vi "Noise_meas.vi"() -> ()   [LabVIEW 2013]
uses:
  <vilib>/DAQmx/read.llb/DAQmx Read (Analog 2D DBL NChan NSamp).vi
  <vilib>/DAQmx/create/channels.llb/DAQmx Create Channel (AI-Voltage-Basic).vi
  <vilib>/DAQmx/configure/timing.llb/DAQmx Timing (Sample Clock).vi
  <vilib>/Analysis/2dsp.llb/1D Cross Correlation (DBL).vi
  <vilib>/DAQmx/miscellaneous.llb/DAQmx Fill In Error Info.vi
  <vilib>/express/express analysis/Spectral/Block/exnSpectralBlock spectral measurements RMS poly.vi
  <vilib>/express/express analysis/Spectral/Block/exnSpectralBlock spectral measurements RMS WFM.vi
  <vilib>/express/express analysis/Spectral/Block/exnSpectralBlock spectral measurements RMS array WFM.vi
  <vilib>/express/express analysis/Spectral/XNode/ExpressSpectralMeasurementsBlockNode.xnode
  <resource>/objmgr/daqmx.rc
  <vilib>/Analysis/NI_AALBase.lvlib
  <vilib>/Analysis/NI_AALPro.lvlib
panel:
  in  "DC1-DC2":tag
  out "Rxy":dbl[](array[numeric])
  out "Waveform Graph 5":dbl[](graph)
  out "dt":dbl
  in  "minimum value 2":dbl=-5.0 format="%0.2f"
  in  "maximum value 2":dbl=5.0 format="%0.2f"
  in  "maximum value":dbl=5.0 format="%0.2f"
  in  "minimum value":dbl=-5.0 format="%0.2f"
  in  "rate":dbl=1000.0 format="%0.2f"
  in  "RF":tag="Dev1/ai0"
  in  "DC2":tag="Dev1/ai2"
  in  "DC1":tag="Dev1/ai1"
  in  "samples per channel":i32=1000
  in  "Tab Control":enum32{"Time", "Spectrum"}(tab)
  out "Waveform Graph":waveform(dbl)[](graph)
  out "Waveform Graph 2":waveform(dbl)[](graph)
  out "Waveform Graph 3":waveform(dbl)(graph)
  out "Waveform Graph 4":waveform(dbl)(graph)
  out "Dc1 Mean":dbl format="%0.2f"
  out "Dc1 Stdev":dbl format="%0.5f"
  out "Dc1 Noise":dbl
  out "Dc2 Noise":dbl
  out "Dc2 Stdev":dbl format="%0.5f"
  out "Dc2 mean":dbl format="%0.2f"
  out "standard deviation 3":dbl format="%0.5f"
  out "mean 3":dbl format="%0.2f"
  out "standard deviation 4":dbl format="%0.5f"
  out "mean 4":dbl format="%0.2f"
  out "mean 5":dbl format="%0.2f"
  out "standard deviation 5":dbl format="%0.5f"
  out "Waveform Graph 9":cluster{"f0":dbl, "df":dbl, "magnitude":dbl[]}[](graph)
  out "Dc2 (mV/V)":cluster{"f0":dbl, "df":dbl, "magnitude":dbl[]}(graph)
  out "Dc1 (mV/V)":cluster{"f0":dbl, "df":dbl, "magnitude":dbl[]}(graph)
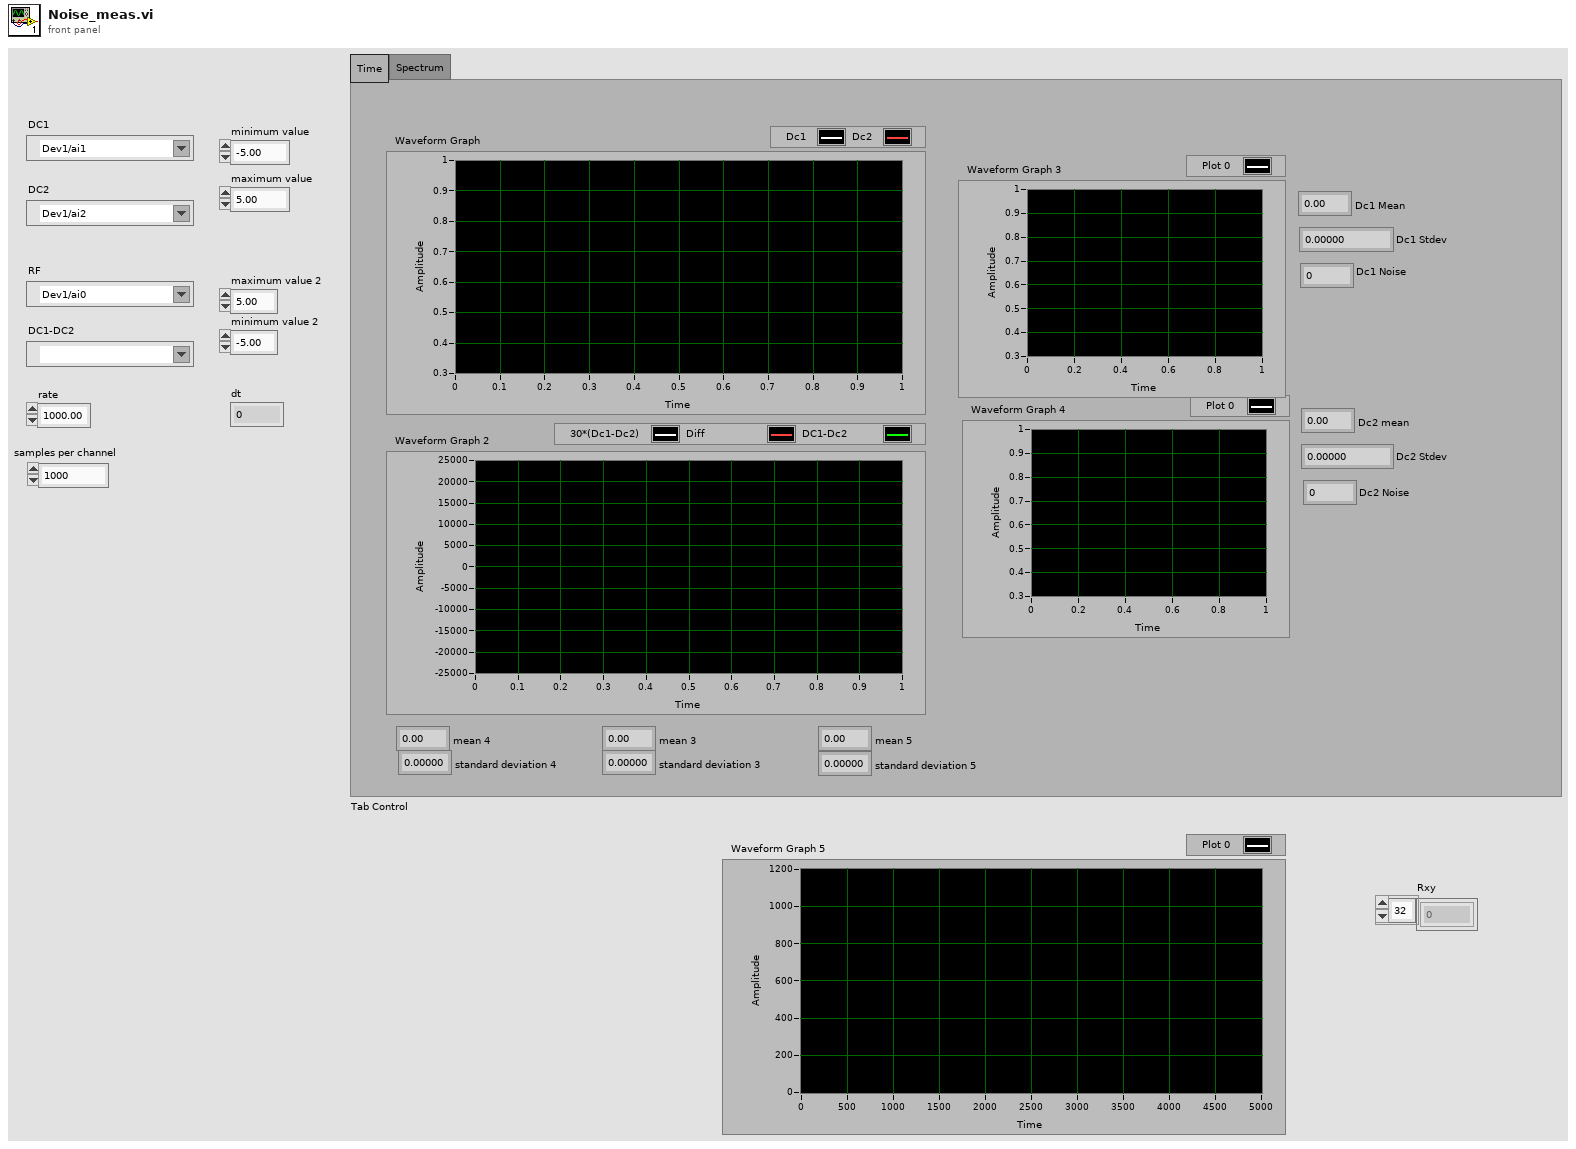
[diagram p1: front panel]
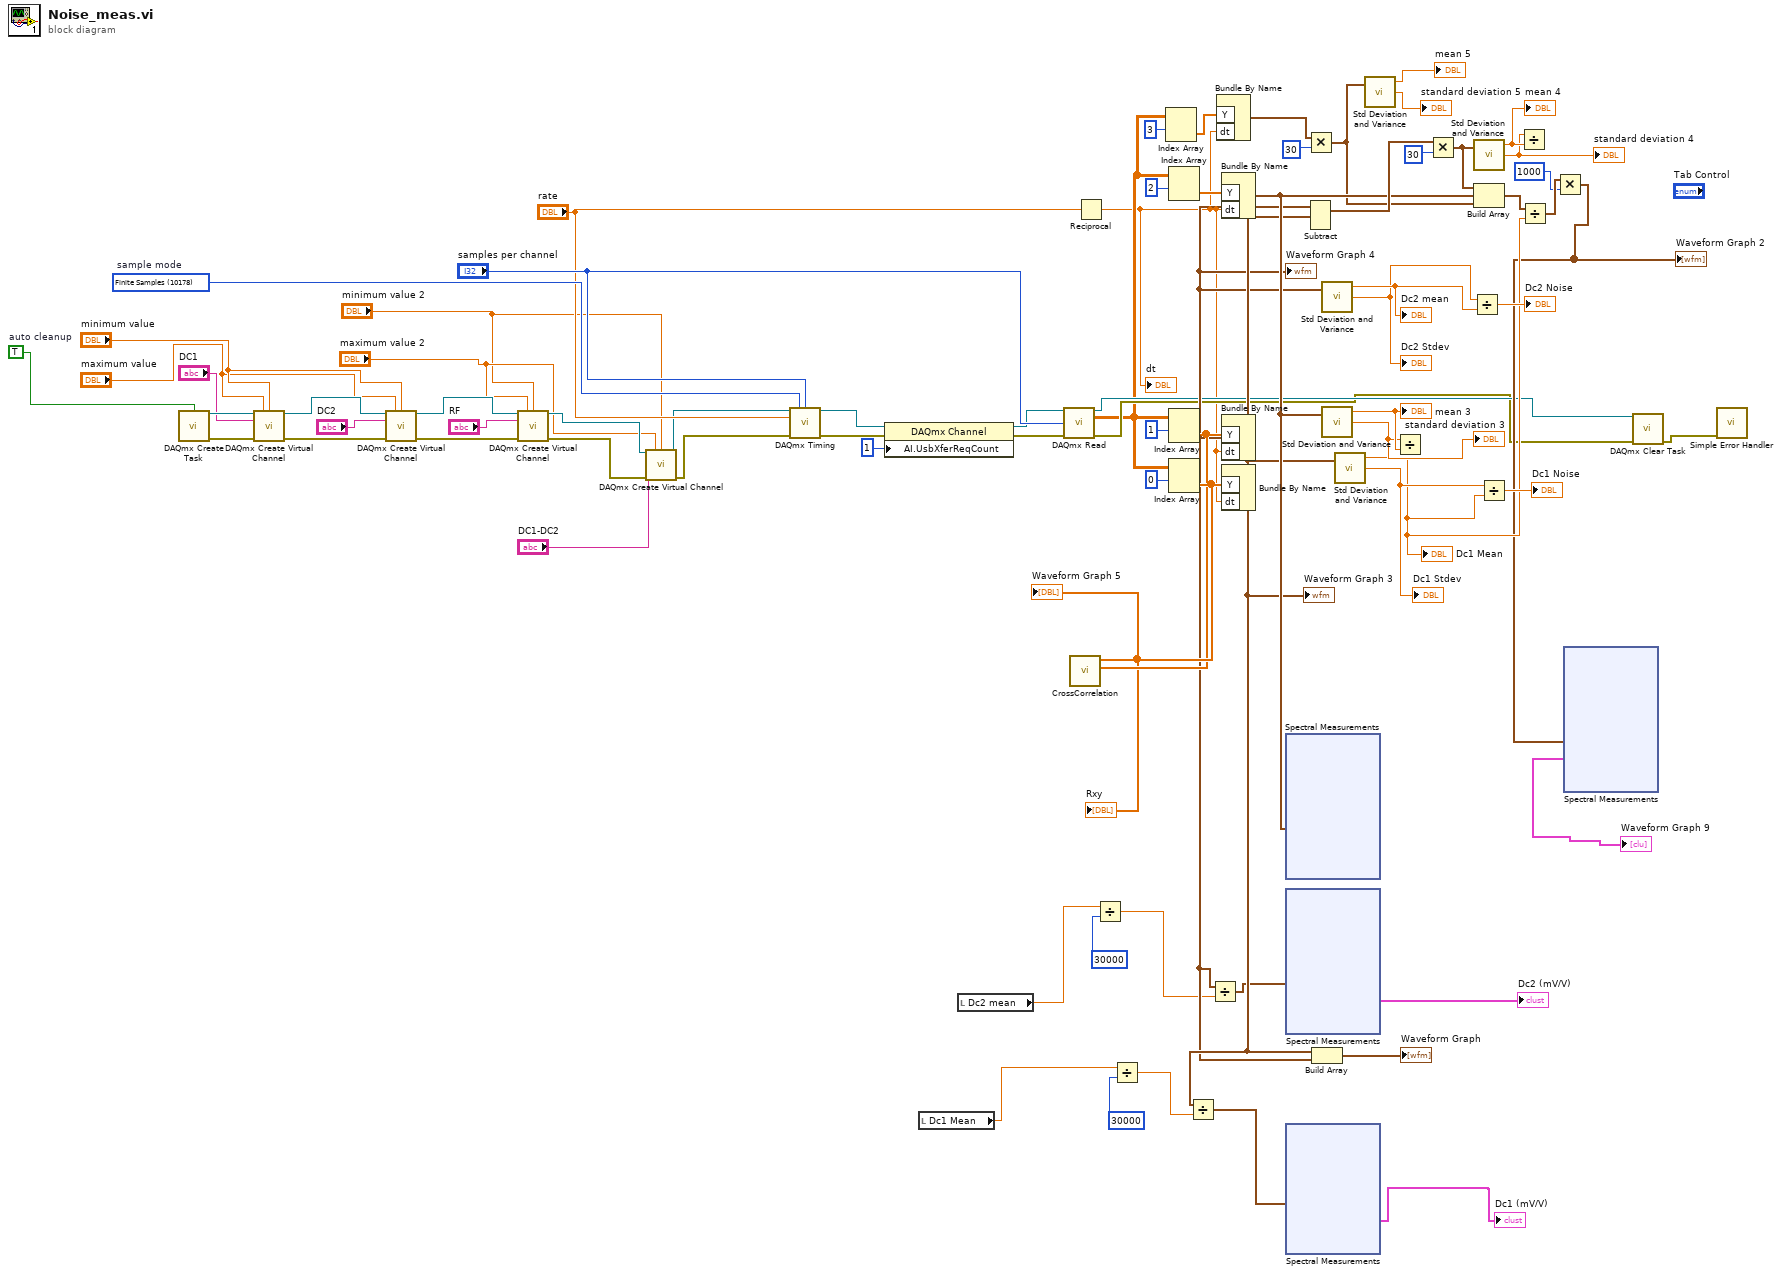
[diagram p0: block diagram]
diagram:
  w75 = 10178 items=["Finite Samples"=10178, "Continuous Samples"=10123, "Hardware Timed Single Point"=12522]  # sample mode
  w78 = TRUE  # auto cleanup
  n1 = call <vilib>:"DAQmx Create Task.vi"("auto cleanup"=w78) -> ("task out"=w72:refnum<k21>, "error out"=w71:errorcluster)  [unwired: 13 in]
  n2 = call-poly <vilib>:"DAQmx Create Virtual Channel.vi"("task in"=w72, "maximum value"="maximum value", "minimum value"="minimum value", "physical channels"="DC1", "error in"=w71) -> ("task out"=w70:refnum<k21>, "error out"=w69:errorcluster)  [unwired: 9 in]
  n3 = call-poly <vilib>:"DAQmx Create Virtual Channel.vi"("task in"=w70, "maximum value"="maximum value", "minimum value"="minimum value", "physical channels"="DC2", "error in"=w69) -> ("task out"=w76:refnum<k21>, "error out"=w77:errorcluster)  [unwired: 9 in]
  n4 = call-poly <vilib>:"DAQmx Create Virtual Channel.vi"("task in"=w76, "maximum value"="maximum value 2", "minimum value"="minimum value 2", "physical channels"="RF", "error in"=w77) -> ("task out"=w14:refnum<k21>, "error out"=w16:errorcluster)  [unwired: 9 in]
  n5 = call-poly <vilib>:"DAQmx Create Virtual Channel.vi"("task in"=w14, "maximum value"="maximum value 2", "minimum value"="minimum value 2", "physical channels"="DC1-DC2", "error in"=w16) -> ("task out"=w13:refnum<k21>, "error out"=w15:errorcluster)  [unwired: 9 in]
  n6 = call-poly <vilib>:"DAQmx Timing.vi"("task/channels in"=w13, "sample mode"=w75, "samples per channel"="samples per channel", "rate"="rate", "error in"=w15) -> ("task out"=w57:refnum<k21>, "error out"=w73:errorcluster)  [unwired: 9 in]
  n7 = property class="DAQmx Channel"(reference=w57, error in=w73, "AI.UsbXferReqCount"=u32 1) -> (reference out=w56:refnum<k21>, error out=w65:errorcluster)
  n8 = local read "Dc1 Mean"() -> (w26:dbl)
  n9 = local read "Dc2 mean"() -> (w29:dbl)
  n10 = call-poly <vilib>:"DAQmx Read.vi"("task/channels in"=w56, "number of samples per channel"="samples per channel", "error in"=w65) -> ("task out"=w19:refnum<k21>, "data"=w9:dbl[][], "error out"=w18:errorcluster)  [unwired: 10 in]
  n11 = Reciprocal(x="rate") -> (1/x=w6:dbl)
  "dt" <- w6
  n12 = Divide(x=w29, y=30000 ("Numeric")) -> (x/y=w28:dbl)
  n13 = Divide(x=w26, y=30000 ("Numeric")) -> (x/y=w25:dbl)
  n14 = Index Array(array=w9, index (row)=3) -> (element=w7:dbl[])  [unwired: 1 in]
  n15 = Index Array(array=w9, index (row)=2) -> (element=w42:dbl[])  [unwired: 1 in]
  n16 = Index Array(array=w9, index (row)=1) -> (element=w39:dbl[])  [unwired: 1 in]
  n17 = Index Array(array=w9, index (row)=0) -> (element=w40:dbl[])  [unwired: 1 in]
  n18 = call-poly <vilib>:"CrossCorrelation.vi"("Y"=w39, "X"=w40) -> ("Rxy"=→"Waveform Graph 5" →"Rxy":dbl[])  [unwired: 8 in, 1 out]
  n19 = Bundle By Name("Y"=w7, "dt"=w6) -> (w4:waveform(dbl))  [unwired: 1 in]
  n20 = Bundle By Name("Y"=w42, "dt"=w6) -> (w41:waveform(dbl))  [unwired: 1 in]
  n21 = Bundle By Name("Y"=w39, "dt"=w6) -> (w33:waveform(dbl))  [unwired: 1 in]
  "Waveform Graph 4" <- w33
  n22 = Divide(x=w33, y=w28) -> (x/y=w32:waveform(dbl))
  n23 = Bundle By Name("Y"=w40, "dt"=w6) -> (w34:waveform(dbl))  [unwired: 1 in]
  "Waveform Graph 3" <- w34
  n24 = Divide(x=w34, y=w25) -> (x/y=w31:waveform(dbl))
  n25 = xnode "Spectral Measurements"("Signals"=w41) -> ()  [unwired: 1 in, 3 out]
  n26 = xnode "Spectral Measurements"("Signals"=w32) -> ("FFT - (RMS)"=→"Dc2 (mV/V)":cluster{"f0":dbl, "df":dbl, "magnitude":dbl[]})  [unwired: 1 in, 2 out]
  n27 = xnode "Spectral Measurements"("Signals"=w31) -> ("FFT - (RMS)"=→"Dc1 (mV/V)":cluster{"f0":dbl, "df":dbl, "magnitude":dbl[]})  [unwired: 1 in, 2 out]
  n28 = Subtract(1:w34, 2:w33) -> (0:w59:waveform(dbl))  [unwired: 1 in, 1 out]
  n29 = Multiply(x=w4, y=30 ("Waveform")) -> (x*y=w3:waveform(dbl))
  n30 = Build Array(w34, w33) -> (→"Waveform Graph":waveform(dbl)[])
  n31 = call <vilib>:"Std Deviation and Variance.vi"("X"=w33) -> ("mean"=w53:dbl, "standard deviation"=w52:dbl)  [unwired: 1 in, 1 out]
  "Dc2 mean" <- w53
  "Dc2 Stdev" <- w52
  n32 = call <vilib>:"Std Deviation and Variance.vi"("X"=w41) -> ("mean"=w51:dbl, "standard deviation"=w50:dbl)  [unwired: 1 in, 1 out]
  "mean 3" <- w51
  "standard deviation 3" <- w50
  n33 = call <vilib>:"Std Deviation and Variance.vi"("X"=w34) -> ("mean"=w36:dbl, "standard deviation"=w55:dbl)  [unwired: 1 in, 1 out]
  "Dc1 Mean" <- w36
  "Dc1 Stdev" <- w55
  n34 = call <vilib>:"Std Deviation and Variance.vi"("X"=w3) -> ("mean"=→"mean 5":dbl, "standard deviation"=→"standard deviation 5":dbl)  [unwired: 1 in, 1 out]
  n35 = Divide(x=w50, y=w51) -> ()  [unwired: 1 out]
  n36 = Multiply(x=w59, y=30 ("Waveform")) -> (x*y=w49:waveform(dbl))
  n37 = Divide(x=w52, y=w53) -> (x/y=→"Dc2 Noise":dbl)
  n38 = call <vilib>:"Std Deviation and Variance.vi"("X"=w49) -> ("mean"=w48:dbl, "standard deviation"=w47:dbl)  [unwired: 1 in, 1 out]
  "mean 4" <- w48
  "standard deviation 4" <- w47
  n39 = Build Array(w49, w41, w3) -> (w37:waveform(dbl)[])
  n40 = Divide(x=w55, y=w36) -> (x/y=→"Dc1 Noise":dbl)
  n41 = Divide(x=w47, y=w48) -> ()  [unwired: 1 out]
  n42 = Divide(x=w37, y=w36) -> (x/y=w21:waveform(dbl)[])
  n43 = Multiply(x=w21, y=1000 ("Numeric")) -> (x*y=w22:waveform(dbl)[])
  "Waveform Graph 2" <- w22
  n44 = xnode "Spectral Measurements"("Signals"=w22) -> ("FFT - (RMS)"=→"Waveform Graph 9":cluster{"f0":dbl, "df":dbl, "magnitude":dbl[]}[])  [unwired: 1 in, 2 out]
  n45 = call <vilib>:"DAQmx Clear Task.vi"("task in"=w19, "error in"=w18) -> ("error out"=w17:errorcluster)  [unwired: 13 in]
  n46 = call <vilib>:"Simple Error Handler.vi"("error in (no error)"=w17) -> ()  [unwired: 4 in, 5 out]
